vi "random circle opg 4.2.vi"() -> ()   [LabVIEW 2015]
panel:
  out "XY Circle Graph":cluster{dbl[], dbl[]}(graph)
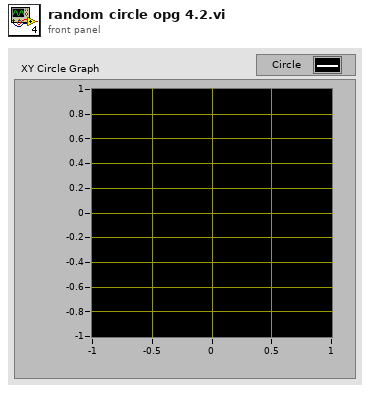
[diagram p1: front panel]
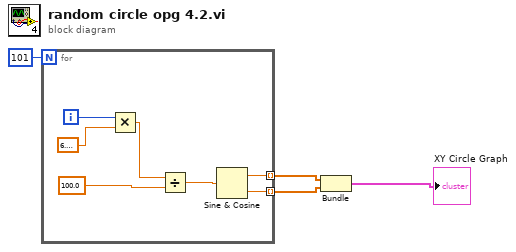
[diagram p0: block diagram]
diagram:
  n1 = for {
    N: 101 -> [_]
    tunnel: [w6] -> w4 mode=indexing
    tunnel: [w5] -> w3 mode=indexing
    i -> [w11]
    n2 = Multiply(x=w11, y=6.283185307179586) -> (x*y=w8:dbl)
    n3 = Divide(x=w8, y=100.0) -> (x/y=w7:dbl)
    n4 = Sine & Cosine(0:w7) -> (1:w6:dbl, 2:w5:dbl)
  }
  n5 = Bundle(w4, w3) -> (→"XY Circle Graph":cluster{dbl[], dbl[]})  [unwired: 1 in]
